vi "FFT e Detecção de frequências.vi"() -> ()   [LabVIEW 2014]
uses:
  <vilib>/express/express analysis/Spectral/XNode/ExpressSpectralMeasurementsBlockNode.xnode
  <vilib>/express/express analysis/Spectral/Block/exnSpectralBlock spectral measurements peak poly.vi
  <vilib>/express/express analysis/Spectral/Block/exnSpectralBlock spectral measurements peak DDT.vi
panel:
  in  "Pattern":string="*.luca"
  out "Formantes encontrados nos arquivos":T1(array[cluster])
  in  "Threshold":dbl=0.001 format="%#_6p"
  in  "Abrir":bool
  out "FFT":dynamicdata(graph)
  in  "Pasta":path=path "/home/lvuser/natinst/bin"
  in  "Caminho no MyRIO":path=path "/home/lvuser/natinst/bin/Aula.txt"
  out "Arquivos encontrados na pasta":string[](array[string])
  in  "Index":i32
  out "Array":dynamicdata[](array[waveform])
  out "Sinal Gravado":dynamicdata(graph)
  in  "On Line":bool
  in  "Gravar":bool
  out "Formantes":cluster{"X":dbl, "Y":dbl}[](graph)
  out "Sinal no Tempo":dynamicdata(graph)
  in  "Stop Button":bool
  # "Pasta para abrir arquivos do MyRIO"
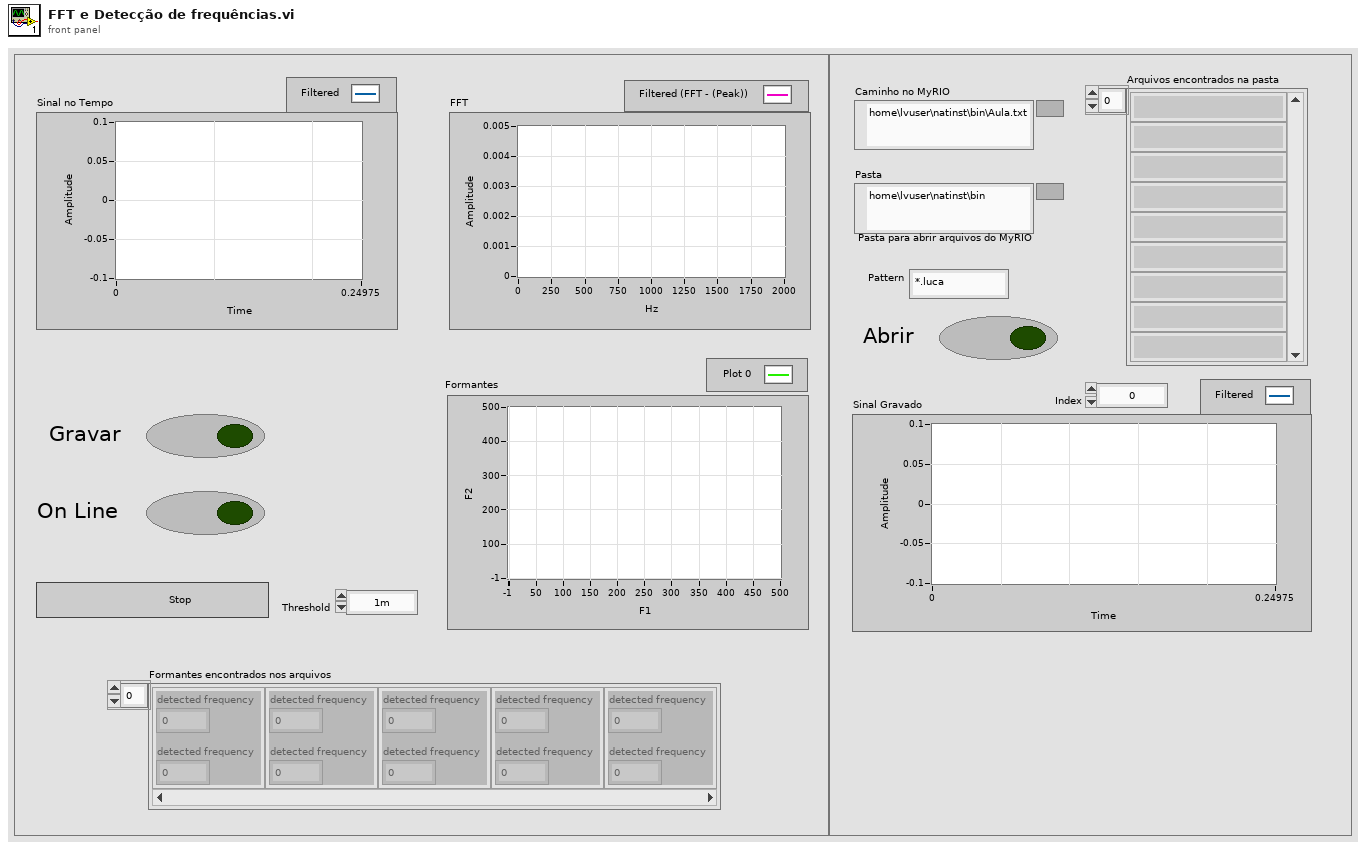
[diagram p1: front panel]
types:
  T1 = cluster{"detected frequency":dbl, "detected frequency":dbl}[]
  T2 = cluster{"averaging mode":u16, "weighting mode":u16, "number of averages":u32}
  T3 = cluster{"dB On (F)":bool, "unwrap phase (F)":bool, "convert to degree (F)":bool}
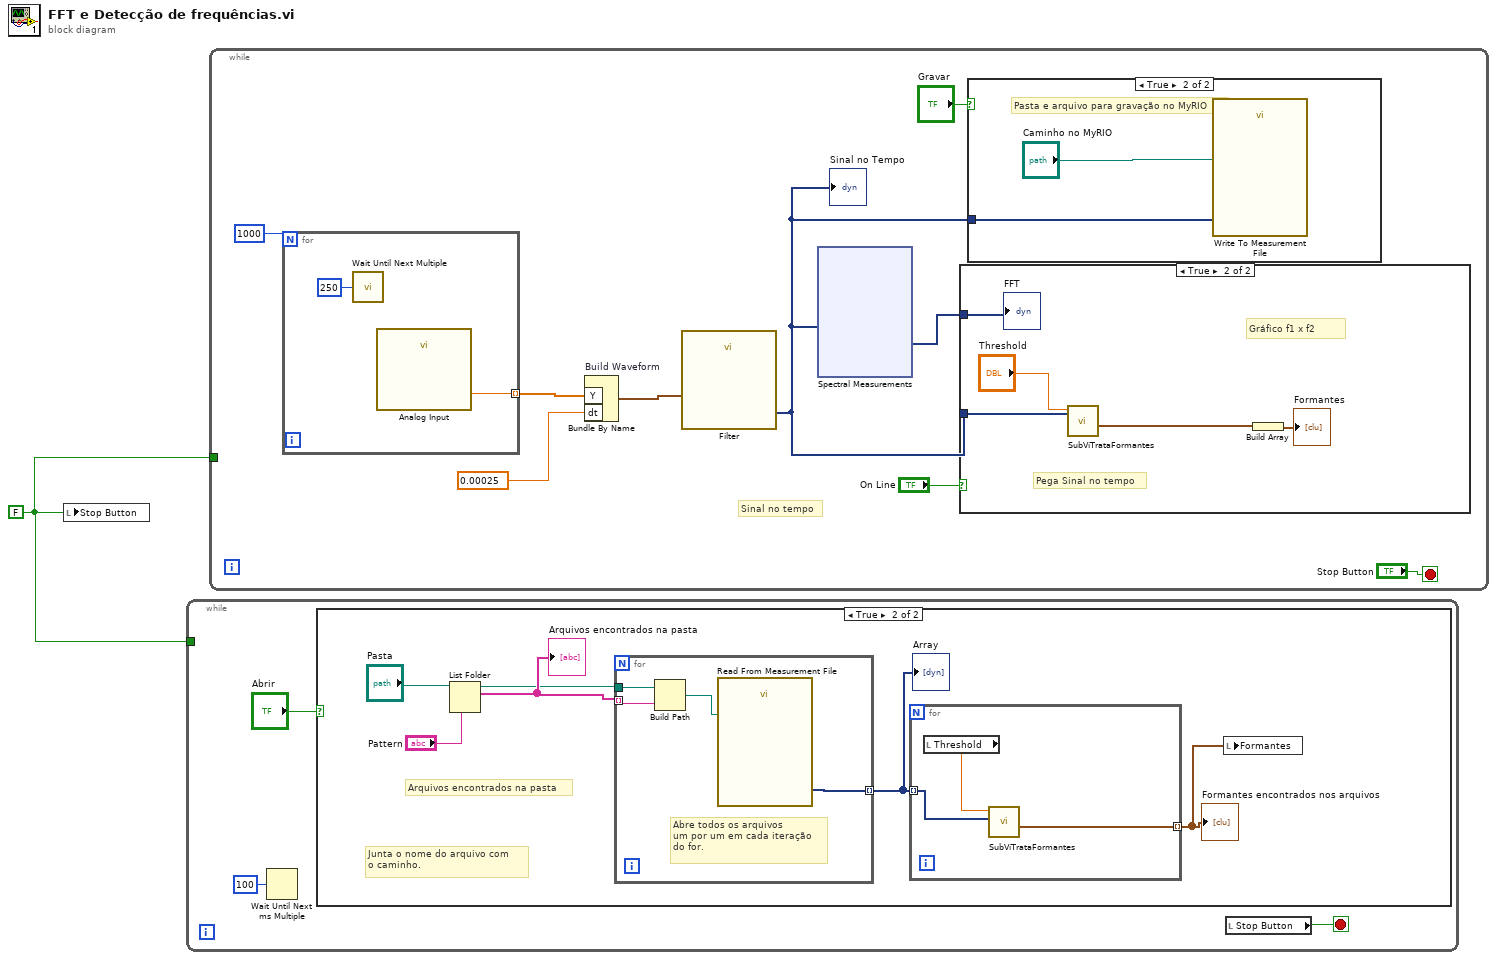
[diagram p0: block diagram]
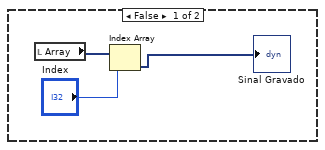
[diagram p2: hidden frame]
diagram:
  w1 = FALSE ("Stop Button")
  n1 = local write "Stop Button"(w1) -> ()
  n2 = while {
    tunnel: w1 -> [_]
    stop <- w4 stop-if-true
    n3 = Wait Until Next ms Multiple(millisecond multiple=u32 100) -> ()  [unwired: 1 out]
    n4 = case shown="True" "Abrir" {
      frame False {
        n5 = local read "Array"() -> (w7:dynamicdata[])
        n6 = Index Array(array=w7, index="Index") -> (element=→"Sinal Gravado":dynamicdata)
      }
      frame True {
        # "Junta o nome do arquivo com\no caminho."
        # "Arquivos encontrados na pasta"
        n7 = List Folder(path="Pasta", pattern="Pattern") -> (path out=w11:path, filenames=w12:string[])  [unwired: 2 in, 2 out]
        "Arquivos encontrados na pasta" <- w12
        n8 = for {
          tunnel: w12 -> [w20] mode=indexing
          tunnel: w11 -> [w19]
          tunnel: [w17] -> w10 mode=indexing
          # "Abre todos os arquivos \num por um em cada iteração\ndo for."
          n9 = Build Path(base path=w19, name or relative path=w20) -> (appended path=w18:path)
          n10 = call "Read From Measurement File"("Filename"=w18) -> ("Signals"=w17:dynamicdata)  [unwired: 5 in, 5 out]
        }
        "Array" <- w10
        n11 = for {
          tunnel: w10 -> [w16] mode=indexing
          tunnel: [w14] -> w8 mode=indexing
          n12 = local read "Threshold"() -> (w15:dbl)
          n13 = call "SubViTrataFormantes.vi"("Filtered Signal"=w16, "Threshold"=w15) -> ("Cluster formantes"=w14:cluster{"F1":dbl, "F2":dbl})  [unwired: 7 in, 2 out]
        }
        "Formantes encontrados nos arquivos" <- w8
        n14 = local write "Formantes"(w8) -> ()
      }
    }
    n15 = local read "Stop Button"() -> (w4:bool)
  }
  n16 = while {
    tunnel: w1 -> [_]
    stop <- "Stop Button" stop-if-true
    # "Sinal no tempo"
    n17 = for {
      N: 1000 ("Numeric") -> [_]
      tunnel: [w47] -> w28 mode=indexing
      n18 = call "Wait Until Next Multiple"("Count(uSec)"=u32 250) -> ()  [unwired: 1 out]
      n19 = call "Analog Input"() -> ("AudioIn/Left"=w47:dbl)  [unwired: 26 in, 1 out]
    }
    n20 = Bundle By Name "Build Waveform"("Y"=w28, "dt"=0.00025) -> (w23:waveform(dbl))  [unwired: 1 in]
    n21 = call "Filter"("Signal"=w23) -> ("Filtered Signal"=w21:dynamicdata)  [unwired: 9 in, 1 out]
    "Sinal no Tempo" <- w21
    n22 = xnode "Spectral Measurements"("Signals"=w21) -> ("FFT - (Peak)"=w22:dynamicdata)  [unwired: 1 in, 2 out]
    n23 = case shown="True" "On Line" {
      tunnel: w22 -> [_ w31]
      tunnel: w21 -> [_ w33]
      frame False {
      }
      frame True {
        # "Pega Sinal no tempo"
        # "Gráfico f1 x f2"
        n24 = call "SubViTrataFormantes.vi"("Filtered Signal"=w33, "Threshold"="Threshold") -> ("Cluster formantes"=w34:cluster{"F1":dbl, "F2":dbl})  [unwired: 7 in, 2 out]
        n25 = Build Array(w34) -> (→"Formantes":cluster{"F1":dbl, "F2":dbl}[])
        "FFT" <- w31
      }
    }
    n26 = case shown="True" "Gravar" {
      tunnel: w21 -> [_ w35]
      frame False {
      }
      frame True {
        # "Pasta e arquivo para gravação no MyRIO"
        n27 = call "Write To Measurement File"("Signals"=w35, "Filename"="Caminho no MyRIO") -> ()  [unwired: 15 in, 3 out]
      }
    }
  }
